vi "Construct_Optimal_Subtrack_(11)-1.vi"(6 "[IN] Indexes for Jumps":i32[](array[numeric]), 8 "error IN":errorcluster, 9 "[IN] Index of recon\nstructed tracks":i32, 10 "[IN] Clusters for Re\nconstructed Tracks":T1, 11 "[IN] Still connected\ntracks in group":T2) -> (0 "error OUT":errorcluster, 2 "[OUT] Clusters for Re\nconstructed Tracks":T1)   [LabVIEW 2013]
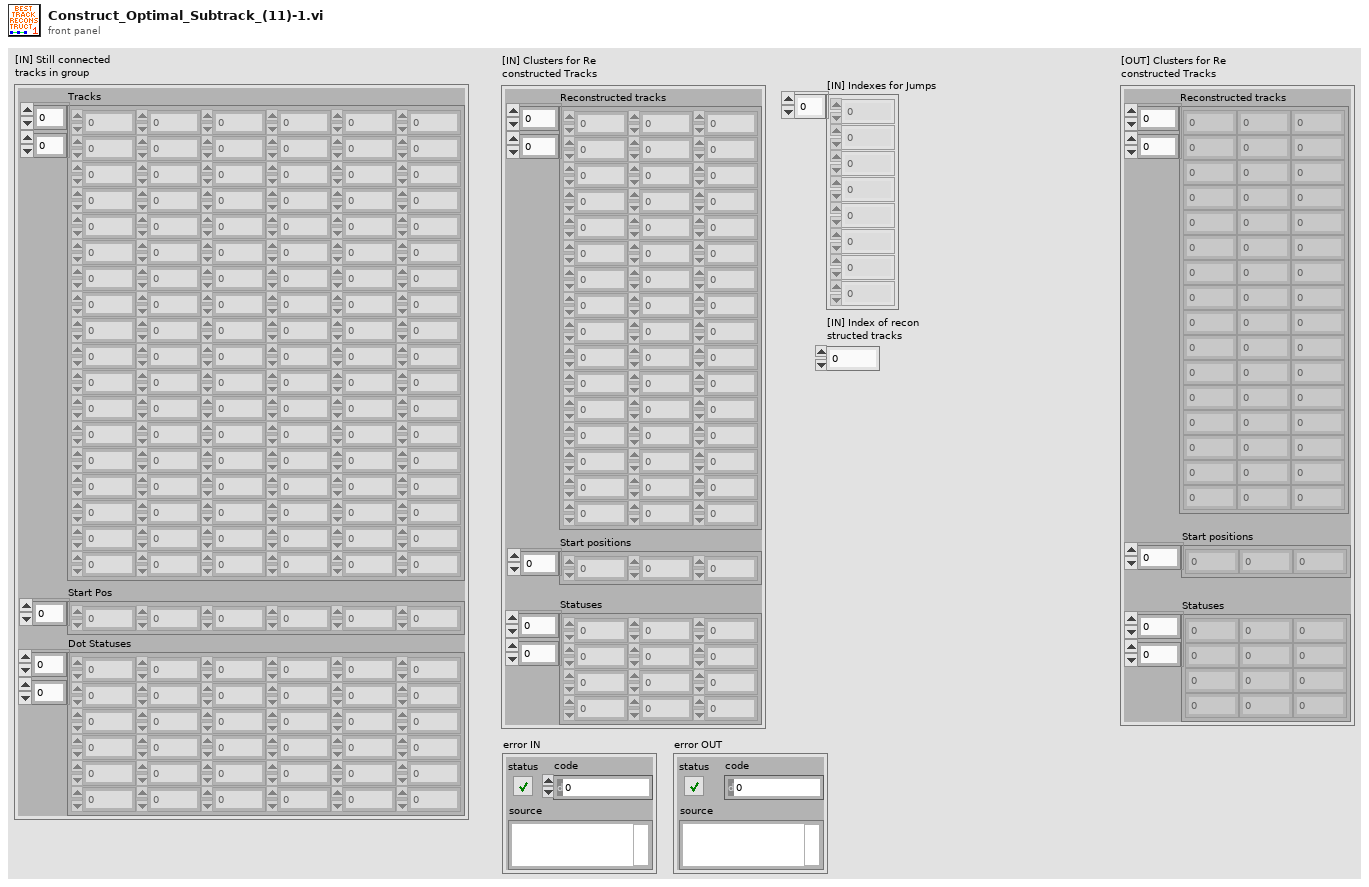
[diagram p1: front panel]
types:
  T1 = cluster{"Reconstructed tracks":dbl[][], "Start positions":i32[], "Statuses":i16[][]}
  T2 = cluster{"Tracks":dbl[][], "Start Pos":i32[], "Dot Statuses":i16[][]}
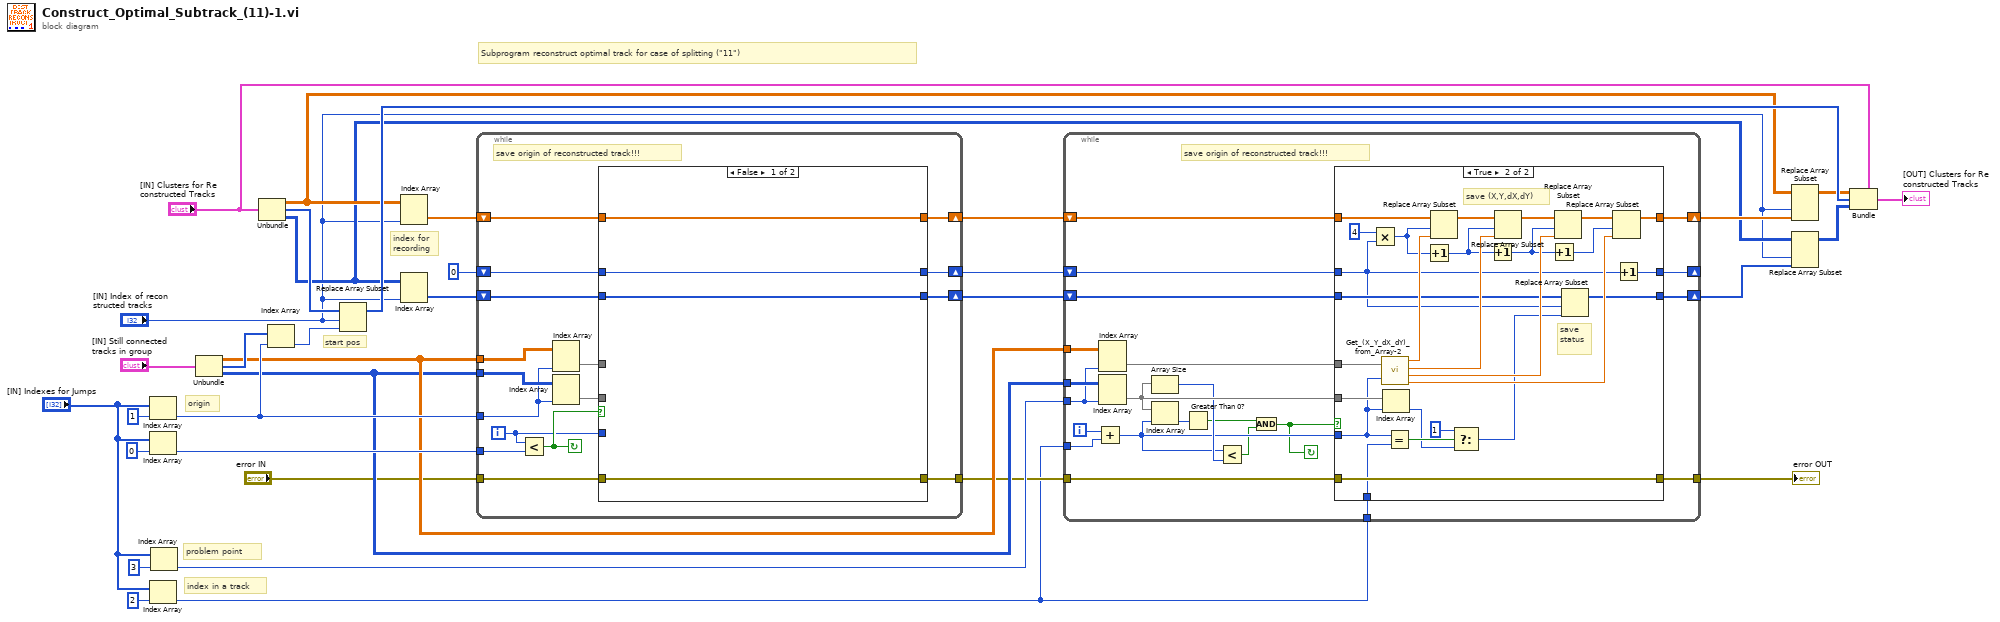
[diagram p0: block diagram]
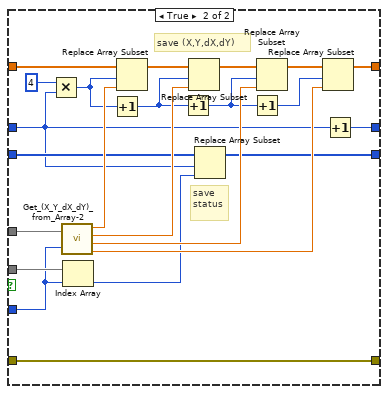
[diagram p3: hidden frame]
diagram:
  # "index in a track"
  # "problem point"
  # "origin"
  # "Subprogram reconstruct optimal track for case of splitting (\"11\")"
  # "index for\nrecording"
  # "start pos"
  n1 = Index Array(array="[IN] Indexes for Jumps", index=1) -> (element=w25:i32)
  n2 = Index Array(array="[IN] Indexes for Jumps", index=0) -> (element=w28:i32)
  n3 = Index Array(array="[IN] Indexes for Jumps", index=2) -> (element=w1:i32)
  n4 = Index Array(array="[IN] Indexes for Jumps", index=3) -> (element=w15:i32)
  n5 = Unbundle("[IN] Still connected\ntracks in group") -> ("Tracks"=w17:dbl[][], "Start Pos"=w26:i32[], "Dot Statuses"=w16:i16[][])
  n6 = Unbundle("[IN] Clusters for Re\nconstructed Tracks") -> ("Reconstructed tracks"=w12:dbl[][], "Start positions"=w27:i32[], "Statuses"=w9:i16[][])
  n7 = Index Array(array=w26, index=w25) -> (element=w24:i32)
  n8 = Replace Array Subset(array=w27, new element=w24, index="[IN] Index of recon\nstructed tracks") -> (w13:i32[])
  n9 = Index Array(array=w12, index (col)="[IN] Index of recon\nstructed tracks") -> (element=w23:dbl[])  [unwired: 1 in]
  n10 = Index Array(array=w9, index (col)="[IN] Index of recon\nstructed tracks") -> (element=w22:i16[])  [unwired: 1 in]
  n11 = while {
    tunnel: w28 -> [w47]
    tunnel: w17 -> [w50]
    tunnel: w16 -> [w49]
    tunnel: w25 -> [w48]
    shift-right: [w39] -> w20
    shift-left: w23 -> [w45]
    shift-right: [w37] -> w18
    shift-left: w22 -> [w41]
    shift-right: [w38] -> w19
    shift-left: 0 -> [w40]
    tunnel: "error IN" -> [w36]
    tunnel: [w35] -> w3
    i -> [w42]
    stop <- w46 continue-if-true
    # "save origin of reconstructed track!!!"
    n12 = Less?(x=w42, y=w47) -> (x < y?=w46:bool)
    n13 = Index Array(array=w50, index (col)=w48) -> (element=w44:dbl[])  [unwired: 1 in]
    n14 = Index Array(array=w49, index (col)=w48) -> (element=w43:i16[])  [unwired: 1 in]
    n15 = case shown="False" w46 {
      tunnel: w45 -> [w54 w75]
      tunnel: w44 -> [_ w77]
      tunnel: w43 -> [_ w76]
      tunnel: w42 -> [_ w60]
      tunnel: w41 -> [w52 w62]
      tunnel: [w52 w59] -> w37
      tunnel: [w54 w58] -> w39
      tunnel: w40 -> [w53 w57]
      tunnel: [w53 w56] -> w38
      tunnel: w36 -> [w51 w55]
      tunnel: [w51 w55] -> w35
      frame False {
      }
      frame True {
        # "save (X,Y,dX,dY)"
        # "save\nstatus"
        n16 = Multiply(x=4, y=w57) -> (x*y=w71:i32)
        n17 = call "Get_(X_Y_dX_dY)_from_Array-2.vi"("(X,Y,dX,dY)"=w77, "Index of Displacement"=w60) -> ("X"=w73:dbl, "Y"=w70:dbl, "dX"=w67:dbl, "dY"=w63:dbl)
        n18 = Index Array(array=w76, index=w60) -> (element=w61:i16)
        n19 = Increment(x=w71) -> (x+1=w68:i32)
        n20 = Replace Array Subset(array=w75, new element=w73, index=w71) -> (w72:dbl[])
        n21 = Increment(x=w68) -> (x+1=w66:i32)
        n22 = Replace Array Subset(array=w72, new element=w70, index=w68) -> (w69:dbl[])
        n23 = Replace Array Subset(array=w62, new element=w61, index=w57) -> (w59:i16[])
        n24 = Increment(x=w66) -> (x+1=w65:i32)
        n25 = Replace Array Subset(array=w69, new element=w67, index=w66) -> (w64:dbl[])
        n26 = Replace Array Subset(array=w64, new element=w63, index=w65) -> (w58:dbl[])
        n27 = Increment(x=w57) -> (x+1=w56:i32)
      }
    }
  }
  n28 = while {
    tunnel: w17 -> [w99]
    tunnel: w16 -> [w98]
    tunnel: w15 -> [w97]
    shift-right: [w92] -> w11
    shift-left: w20 -> [w96]
    shift-right: [w90] -> w8
    shift-left: w18 -> [w94]
    shift-right: [w91] -> _
    shift-left: w19 -> [w93]
    tunnel: w1 -> [w88]
    tunnel: w3 -> [w80]
    tunnel: [w79] -> w2
    tunnel: w1 -> [w78]
    i -> [w89]
    stop <- w81 continue-if-true
    # "save origin of reconstructed track!!!"
    n29 = Add(x=w89, y=w88) -> (x+y=w84:i32)
    n30 = Index Array(array=w99, index (col)=w97) -> (element=w95:dbl[])  [unwired: 1 in]
    n31 = Index Array(array=w98, index (col)=w97) -> (element=w87:i16[])  [unwired: 1 in]
    n32 = Array Size(array=w87) -> (size(s)=w85:i32)
    n33 = Index Array(array=w87, index=w84) -> (element=w86:i16)
    n34 = Greater Than 0?(x=w86) -> (x > 0?=w83:bool)
    n35 = Less?(x=w84, y=w85) -> (x < y?=w82:bool)
    n36 = And(x=w83, y=w82) -> (x .and. y?=w81:bool)
    n37 = case shown="True" w81 {
      tunnel: w96 -> [w103 w128]
      tunnel: w95 -> [_ w130]
      tunnel: w87 -> [_ w129]
      tunnel: w84 -> [_ w109]
      tunnel: w94 -> [w101 w115]
      tunnel: [w101 w114] -> w90
      tunnel: [w103 w113] -> w92
      tunnel: w93 -> [w102 w112]
      tunnel: [w102 w111] -> w91
      tunnel: w80 -> [w100 w110]
      tunnel: [w100 w110] -> w79
      tunnel: w78 -> [_ w108]
      frame False {
      }
      frame True {
        # "save (X,Y,dX,dY)"
        # "save\nstatus"
        n38 = Multiply(x=4, y=w112) -> (x*y=w124:i32)
        n39 = call "Get_(X_Y_dX_dY)_from_Array-2.vi"("(X,Y,dX,dY)"=w130, "Index of Displacement"=w109) -> ("X"=w126:dbl, "Y"=w123:dbl, "dX"=w120:dbl, "dY"=w116:dbl)
        n40 = Index Array(array=w129, index=w109) -> (element=w106:i16)
        n41 = Equal?(x=w109, y=w108) -> (x = y?=w107:bool)
        n42 = Increment(x=w124) -> (x+1=w121:i32)
        n43 = Replace Array Subset(array=w128, new element=w126, index=w124) -> (w125:dbl[])
        n44 = Select(t=i16 1, s=w107, f=w106) -> (s? t:f=w104:i16)
        n45 = Increment(x=w121) -> (x+1=w119:i32)
        n46 = Replace Array Subset(array=w125, new element=w123, index=w121) -> (w122:dbl[])
        n47 = Increment(x=w119) -> (x+1=w118:i32)
        n48 = Replace Array Subset(array=w122, new element=w120, index=w119) -> (w117:dbl[])
        n49 = Replace Array Subset(array=w115, new element=w104, index=w112) -> (w114:i16[])
        n50 = Replace Array Subset(array=w117, new element=w116, index=w118) -> (w113:dbl[])
        n51 = Increment(x=w112) -> (x+1=w111:i32)
      }
    }
  }
  "error OUT" <- w2
  n52 = Replace Array Subset(array=w12, new element=w11, index (col)="[IN] Index of recon\nstructed tracks") -> (w10:dbl[][])  [unwired: 1 in]
  n53 = Replace Array Subset(array=w9, new element=w8, index (col)="[IN] Index of recon\nstructed tracks") -> (w6:i16[][])  [unwired: 1 in]
  n54 = Bundle(cluster="[IN] Clusters for Re\nconstructed Tracks", "Reconstructed tracks"=w10, "Start positions"=w13, "Statuses"=w6) -> (→"[OUT] Clusters for Re\nconstructed Tracks":T1)
